vi "test-UKF-test1-callback.vi"(9 "U":T1, 10 "X":T1, 11 "Variant":variant) -> (0 "Error":bool, 3 "Return":T1)   [LabVIEW 2019]
uses:
  <vilib>/Analysis/Matrix/Datatypes/RealMatrix.ctl
  <vilib>/Analysis/baseanly.llb/Real A x B.vi
  <vilib>/Rock Robotics/WPI/ThirdParty/JAS_Junk/TrajLib/MatBuilder_Create.vi
  <vilib>/Analysis/NI_AALBase.lvlib
  <vilib>/Rock Robotics/WPI/ThirdParty/JAS_Junk/TrajLib/Trajectory_Library.lvlib
  <vilib>/Analysis/Matrix/NI_Matrix.lvlib
panel:
  # "6, 1"
  # "SIGMAS"
  # "WEIGHTS"
  # "2, 1"
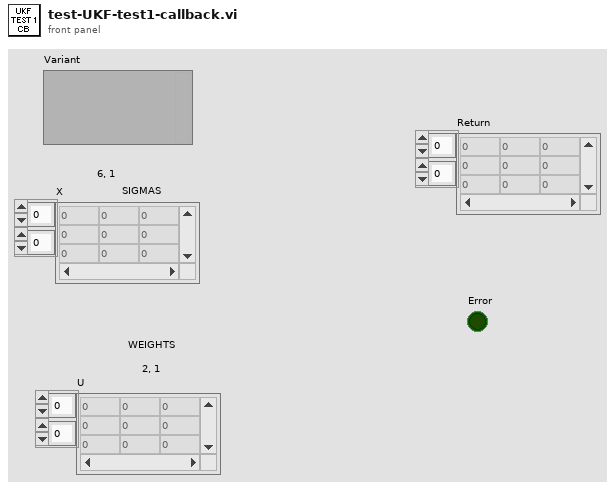
[diagram p1: front panel]
types:
  T1 = typedef "NI_Matrix.lvlib/RealMatrix.ctl" = dbl[][]
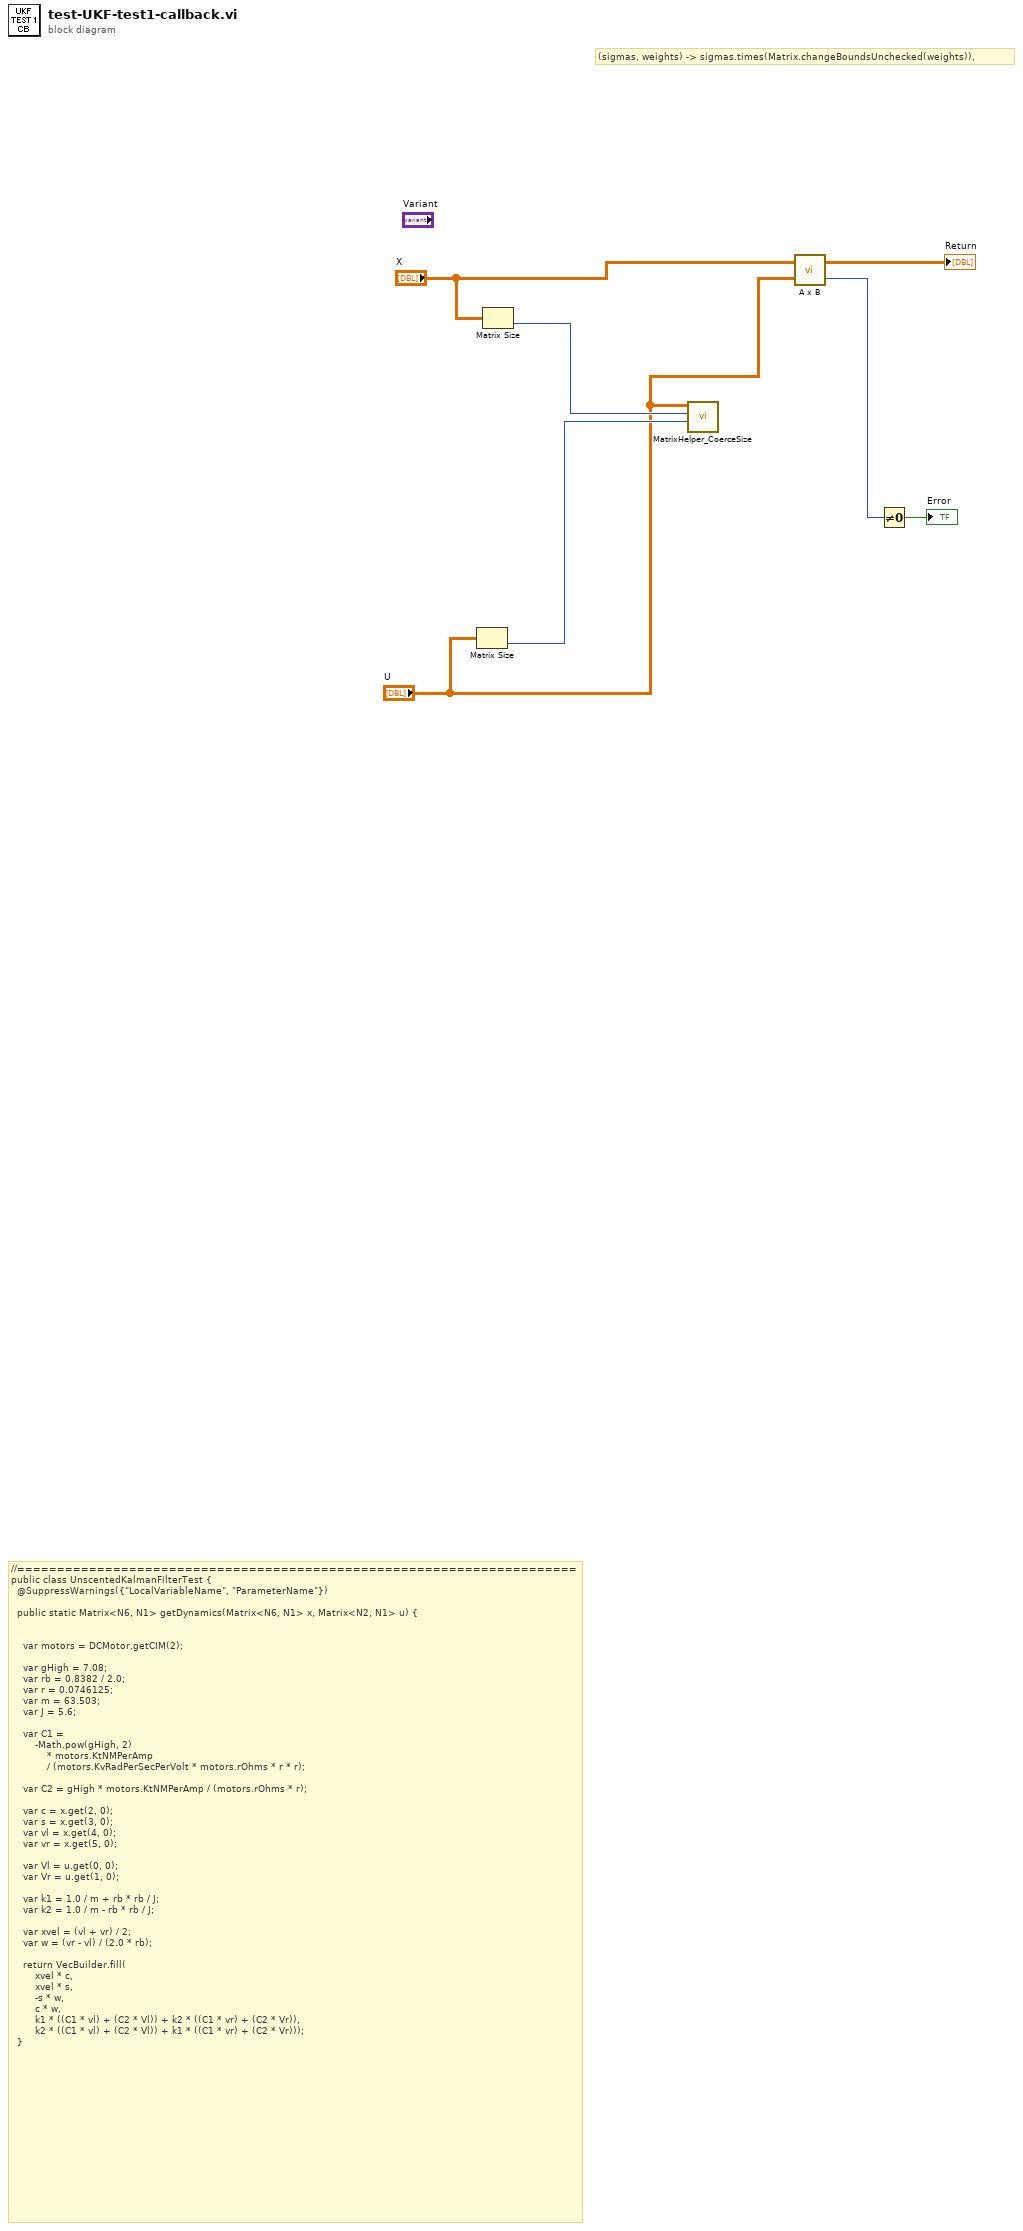
[diagram p0: block diagram]
diagram:
  # "(sigmas, weights) -> sigmas.times(Matrix.changeBoundsUnchecked(weights)),"
  # "//======================================================================\npublic class UnscentedKalmanFilterTest {\n  @SuppressWarnings({\"LocalVariableName\", \"ParameterName\"})\n\n  public static Matrix<N6, N1> getDynamics(Matrix<N6, N1> x, Matrix<N2, N1> u) {\n\n\n    var motors = DCMotor.getCIM(2);\n\n    var gHigh = 7.08;\n    var rb = 0.8382 / 2.0;\n    var r = 0.0746125;\n    var m = 63.503;\n    var J = 5.6;\n\n    var C1 =\n        -Math.pow(gHigh, 2)\n            * motors.KtNMPerAmp\n            / (motors.KvRadPerSecPerVolt * motors.rOhms * r * r);\n\n    var C2 = gHigh * motors.KtNMPerAmp / (motors.rOhms * r);\n\n    var c = x.get(2, 0);\n    var s = x.get(3, 0);\n    var vl = x.get(4, 0);\n    var vr = x.get(5, 0);\n\n    var Vl = u.get(0, 0);\n    var Vr = u.get(1, 0);\n\n    var k1 = 1.0 / m + rb * rb / J;\n    var k2 = 1.0 / m - rb * rb / J;\n\n    var xvel = (vl + vr) / 2;\n    var w = (vr - vl) / (2.0 * rb);\n\n    return VecBuilder.fill(\n        xvel * c,\n        xvel * s,\n        -s * w,\n        c * w,\n        k1 * ((C1 * vl) + (C2 * Vl)) + k2 * ((C1 * vr) + (C2 * Vr)),\n        k2 * ((C1 * vl) + (C2 * Vl)) + k1 * ((C1 * vr) + (C2 * Vr)));\n  }"
  n1 = Matrix Size(0:"U") -> (2:w5:i32)  [unwired: 1 out]
  n2 = Matrix Size(0:"X") -> (2:w6:i32)  [unwired: 1 out]
  n3 = call <vilib>:"MatrixHelper_CoerceSize.vi"("Columns"=w5, "Rows"=w6, "input matrix"="U") -> ()  [unwired: 7 in, 2 out]
  n4 = call-poly <vilib>:"A x B.vi"("B"="U", "A"="X") -> ("error"=w3:i32, "A x B"=→"Return":T1)
  n5 = Not Equal To 0?(x=w3) -> (x != 0?=→"Error":bool)
